vi "Run System Exec.vi"(7 "cmdline in error in":bool, 8 "error in":errorcluster, 9 "working directory in":path, 10 "vi name in":string, 11 "command in":string) -> (0 "error out":errorcluster, 2 "standard error out":string, 3 "standard output out":string)   [LabVIEW 2019]
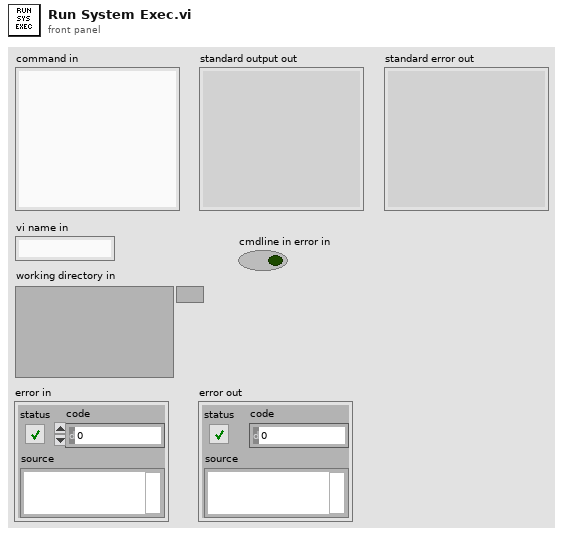
[diagram p1: front panel]
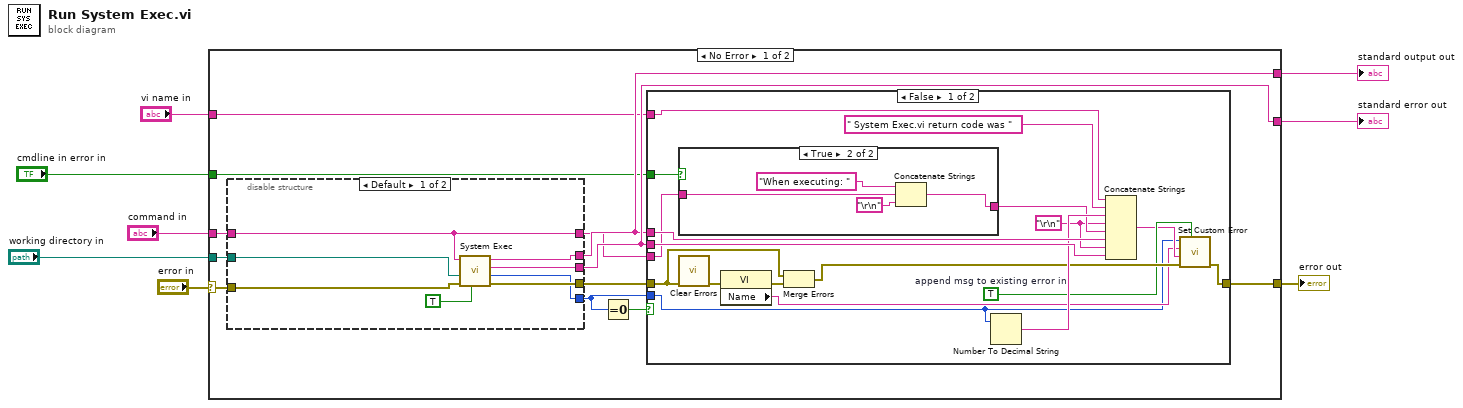
[diagram p0: block diagram]
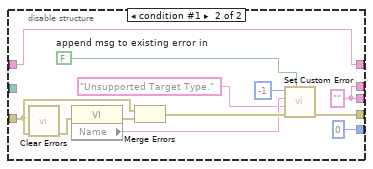
[diagram p2: hidden frame]
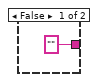
[diagram p3: hidden frame]
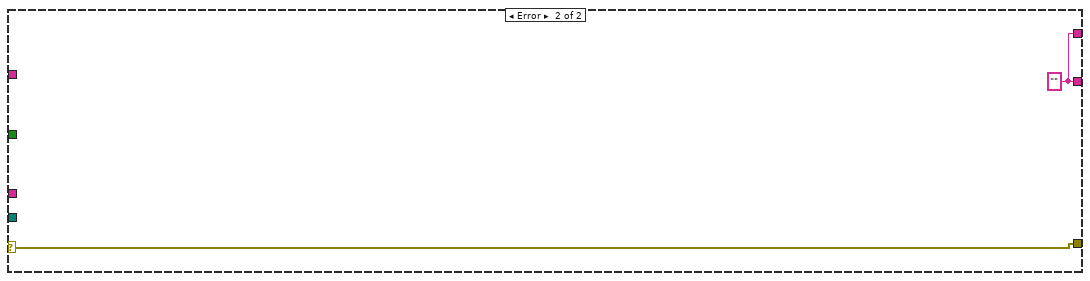
[diagram p5: hidden frame]
diagram:
  n1 = case shown="No Error" "error in" {
    selector: "error in" -> [w15 w66]
    tunnel: "vi name in" -> [w13 _]
    tunnel: [w18 w65] -> w7
    tunnel: [w17 w65] -> w6
    tunnel: "command in" -> [w10 _]
    tunnel: [w16 w66] -> w4
    tunnel: "working directory in" -> [w14 _]
    tunnel: "cmdline in error in" -> [w11 _]
    frame No Error {
      n2 = disable-structure shown="Default" {
        disable-tunnel: [w28 w31] -> w20
        disable-tunnel: [w27 w39] -> w18
        disable-tunnel: [w26 w39] -> w17
        disable-tunnel: w15 -> [w24 w30]
        disable-tunnel: w14 -> [w23 _]
        disable-tunnel: [w22 0 ("return code")] -> w12
        disable-tunnel: w10 -> [w21 w29]
        disable-tunnel: [w21 w29] -> w9
        frame condition #0 (active) {
          n3 = call <vilib>:"System Exec.vi"("run minimized? (F)"=TRUE, "error in (no error)"=w24, "working directory"=w23, "command line"=w21) -> ("error out"=w28:errorcluster, "return code"=w22:i32, "standard error"=w27:string, "standard output"=w26:string)  [unwired: 4 in]
        }
        frame condition #1 {
          w38 = FALSE  # append msg to existing error in
          w39 = "" ("standard output")
          n4 = call <vilib>:"Clear Errors.vi"("error in (no error)"=w30) -> ("error out"=w36:errorcluster)  [unwired: 5 in, 1 out]
          n5 = property class="VI"(error in=w36) -> (error out=w34:errorcluster, "Name"=w33:string)  [unwired: 1 in, 1 out]
          n6 = Merge Errors(w30, w34) -> (w35:errorcluster)
          n7 = call "Set Custom Error.vi"("append msg to existing error in"=w38, "error in"=w35, "message in"="Unsupported Target Type." ("source"), "source in"=w33, "code in"=-1 ("code")) -> ("error out"=w31:errorcluster)  [unwired: 6 in]
        }
      }
      n8 = Equal To 0?(x=w12) -> (x = 0?=w19:bool)
      n9 = case shown="False" w19 {
        tunnel: [w53 w64] -> w16
        tunnel: w20 -> [w46 w64]
        tunnel: w17 -> [w58 _]
        tunnel: w18 -> [w57 _]
        tunnel: w12 -> [w45 _]
        tunnel: w13 -> [w56 _]
        tunnel: w11 -> [w44 _]
        tunnel: w9 -> [w43 _]
        frame False {
          w49 = TRUE  # append msg to existing error in
          w41 = "\r\n"
          n10 = case shown="True" w44 {
            tunnel: w43 -> [_ w62]
            tunnel: ["" w61] -> w42
            frame False {
            }
            frame True {
              n11 = Concatenate Strings("When executing: ", w62, "\r\n") -> (w61:string)
            }
          }
          n12 = call <vilib>:"Clear Errors.vi"("error in (no error)"=w46) -> ("error out"=w52:errorcluster)  [unwired: 5 in, 1 out]
          n13 = property class="VI"(error in=w52) -> (error out=w50:errorcluster, "Name"=w47:string)  [unwired: 1 in, 1 out]
          n14 = Merge Errors(w46, w50) -> (w51:errorcluster)
          n15 = Number To Decimal String(number=w45) -> (decimal integer string=w54:string)  [unwired: 1 in]
          n16 = Concatenate Strings(w56, " System Exec.vi return code was " ("search string/char (-)"), w54, w41, w42, w58, w41, w57) -> (w48:string)
          n17 = call "Set Custom Error.vi"("append msg to existing error in"=w49, "error in"=w51, "message in"=w48, "source in"=w47, "code in"=w45) -> ("error out"=w53:errorcluster)  [unwired: 6 in]
        }
        frame True {
        }
      }
    }
    frame Error {
      w65 = "" ("standard error")
    }
  }
  "standard error out" <- w7
  "standard output out" <- w6
  "error out" <- w4
